vi "Write Range Double.vi"(8 "error in (no error)":errorcluster, 10 "Range Array":T1[](array[typedef]), 11 "Double Scanner in":refnum<class "Double Scanner.lvclass">) -> (0 "error out":errorcluster, 2 "# Points":u32, 3 "Double Scanner out":refnum<class "Double Scanner.lvclass">)   [LabVIEW 2012, in "Double Scanner.lvclass"]
doc: "Set the Range of this Scanner to the Range of another Scanner."
uses:
  Double Scanner.lvclass
  Scanner/Range.ctl
  Double Scanner.lvclass/Double Scanner.ctl
  Scanner/Scanner.lvclass
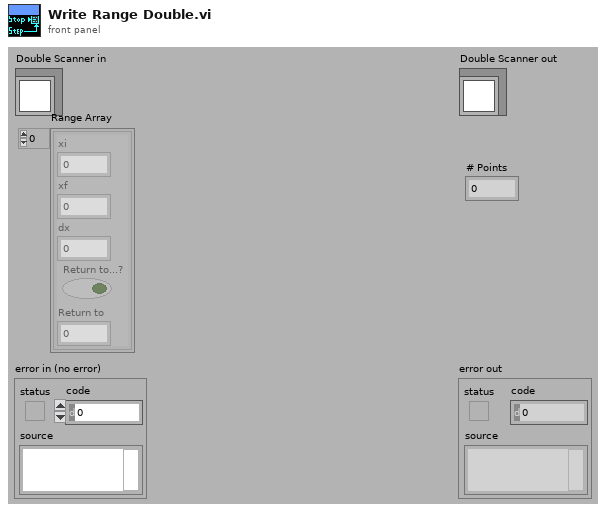
[diagram p1: front panel]
types:
  T1 = typedef "Scanner.lvclass/Range.ctl" = cluster{"xi":dbl, "xf":dbl, "dx":dbl, "Return to...?":bool, "Return to":dbl}
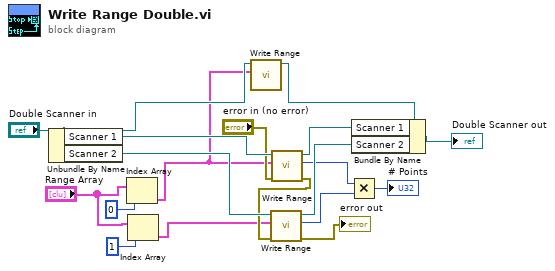
[diagram p0: block diagram]
diagram:
  n1 = Unbundle By Name("Double Scanner in") -> ("Scanner 1"=w9:refnum<class "Scanner.lvclass">, "Scanner 2"=w13:refnum<class "Scanner.lvclass">)
  n2 = Index Array(array="Range Array", index=0) -> (element=w1:T1)
  n3 = Index Array(array="Range Array", index=1) -> (element=w4:T1)
  n4 = call-dynamic "Write Range.vi"("Range"=w1, "Scanner in"="Double Scanner in") -> ("Scanner out"=w2:refnum<class "Double Scanner.lvclass">)  [unwired: 7 in, 2 out]
  n5 = call-dynamic "Write Range.vi"("error in (no error)"="error in (no error)", "Range"=w1, "Scanner in"=w9) -> ("error out"=w7:errorcluster, "# Points"=w6:u32, "Scanner out"=w5:refnum<class "Scanner.lvclass">)  [unwired: 6 in]
  n6 = call-dynamic "Write Range.vi"("error in (no error)"=w7, "Range"=w4, "Scanner in"=w13) -> ("error out"=→"error out":errorcluster, "# Points"=w11:u32, "Scanner out"=w10:refnum<class "Scanner.lvclass">)  [unwired: 6 in]
  n7 = Multiply(x=w6, y=w11) -> (x*y=→"# Points":u32)
  n8 = Bundle By Name(cluster=w2, "Scanner 1"=w5, "Scanner 2"=w10) -> (→"Double Scanner out":refnum<class "Double Scanner.lvclass">)
